vi "Calculation_Velocities_Statistics-3.vi"(8 "error IN":errorcluster, 9 "[IN] Velocities and Times":T3, 10 "[IN] Filtered Tracks":cluster{"Tracks":dbl[], "Start Pos":i32}[](array[cluster]), 11 "[IN] Movie Values":T2 {"Particle Fil Setups"."Type of particle filter"."Measurement Parameter" items=["Center of Mass X", "Center of Mass Y", "First Pixel X", "First Pixel Y", "Bounding Rect Left", "Bounding Rect Top", "Bounding Rect Right", "Bounding Rect Bottom", "Max Feret Diameter Start X", "Max Feret Diameter Start Y", "Max Feret Diameter End X", "Max Feret Diameter End Y", "Max Horiz. Segment Length Left", "Max Horiz. Segment Length Right", "Max Horiz. Segment Length Row", "-", "Bounding Rect Width", "Bounding Rect Height", "Bounding Rect Diagonal", "Perimeter", "Convex Hull Perimeter", "Holes' Perimeter", "Max Feret Diameter", "Equivalent Ellipse Major Axis", "Equivalent Ellipse Minor Axis", "Equivalent Ellipse Minor Axis (Feret)", "Equivalent Rect Long Side", "Equivalent Rect Short Side", "Equivalent Rect Diagonal", "Equivalent Rect Short Side (Feret)", "Average Horiz. Segment Length", "Average Vert. Segment Length", "Hydraulic Radius", "Waddel Disk Diameter", "-", "Area", "Holes' Area", "Particle & Holes' Area", "Convex Hull Area", "Image Area", "-", "Number of Holes", "Number of Horiz. Segments", "Number of Vert. Segments", "-", "Orientation", "Max Feret Diameter Orientation", "-", "% Area/Image Area", "% Area/(Particle & Holes' Area)", "Ratio of Equivalent Ellipse Axes", "Ratio of Equivalent Rect Sides", "-", "Elongation Factor", "Compactness Factor", "Heywood Circularity Factor", "Type Factor", "-", "Sum X", "Sum Y", "Sum XX", "Sum XY", "Sum YY", "Sum XXX", "Sum XXY", "Sum XYY", "Sum YYY", "-", "Moment of Inertia XX", "Moment of Inertia XY", "Moment of Inertia YY", "Moment of Inertia XXX", "Moment of Inertia XXY", "Moment of Inertia XYY", "Moment of Inertia YYY", "Norm. Moment of Inertia XX", "Norm. Moment of Inertia XY", "Norm. Moment of Inertia YY", "Norm. Moment of Inertia XXX", "Norm. Moment of Inertia XXY", "Norm. Moment of Inertia XYY", "Norm. Moment of Inertia YYY", "Hu Moment 1", "Hu Moment 2", "Hu Moment 3", "Hu Moment 4", "Hu Moment 5", "Hu Moment 6", "Hu Moment 7"]}) -> (0 "error OUT":errorcluster, 1 "[OUT] Velocities and Times":T3)   [LabVIEW 2013]
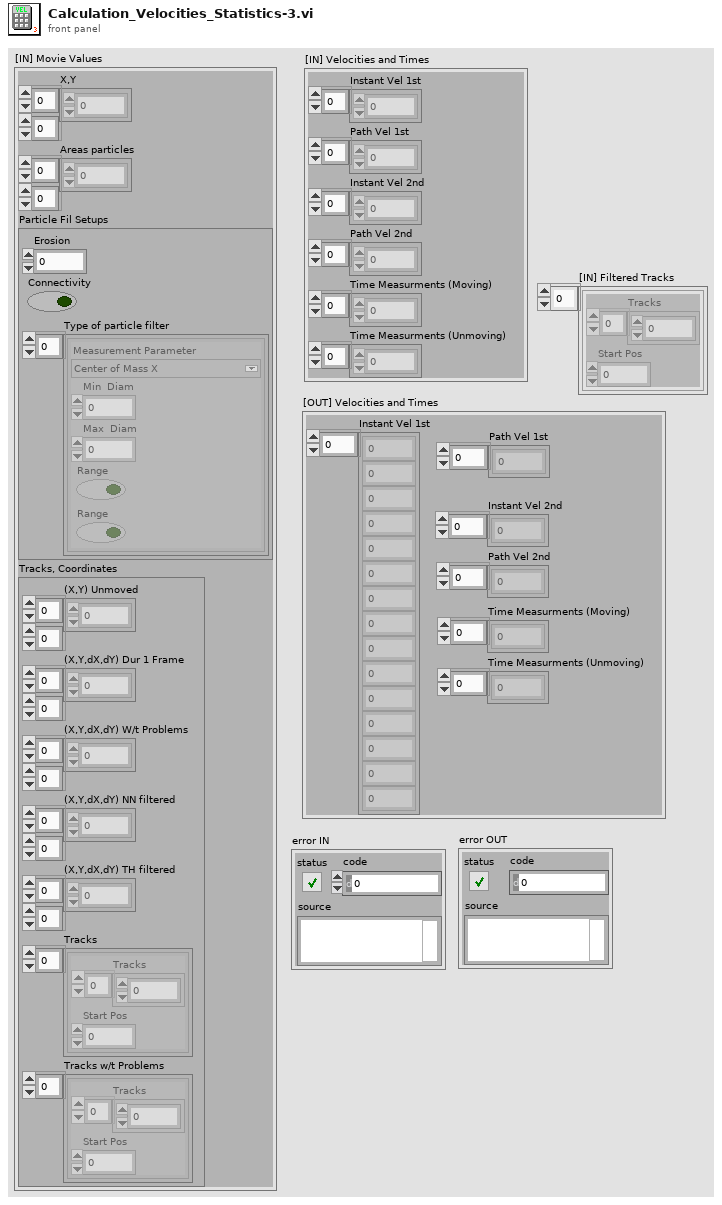
[diagram p1: front panel]
types:
  T1 = typedef "Particle Parameters" = i32
  T2 = cluster{"X,Y":dbl[][], "Areas particles":dbl[][], "Particle Fil Setups":cluster{"Erosion":i32, "Connectivity ":bool, "Type of particle filter":cluster{"Measurement Parameter":T1, "Min  Diam":dbl, "Max  Diam":dbl, "Range":bool, "Range":bool}[]}, "Tracks, Coordinates":cluster{"(X,Y) Unmoved":dbl[][], "(X,Y,dX,dY) Dur 1 Frame":dbl[][], "(X,Y,dX,dY) W/t Problems":dbl[][], "(X,Y,dX,dY) NN filtered":dbl[][], "(X,Y,dX,dY) TH filtered":dbl[][], "Tracks":cluster{"Tracks":dbl[], "Start Pos":i32}[], "Tracks w/t Problems":cluster{"Tracks":dbl[], "Start Pos":i32}[]}}
  T3 = cluster{"Instant Vel 1st":dbl[], "Path Vel 1st ":dbl[], "Instant Vel 2nd  ":dbl[], "Path Vel 2nd":dbl[], "Time Measurments (Moving)":i32[], "Time Measurments (Unmoving) ":i16[]}
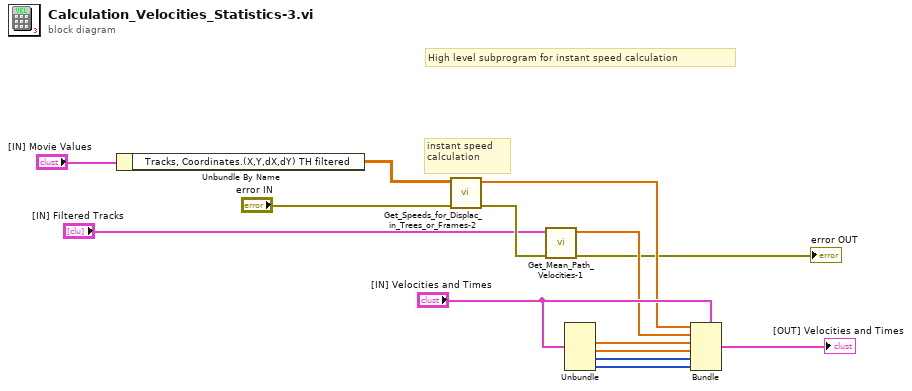
[diagram p0: block diagram]
diagram:
  # "High level subprogram for instant speed calculation"
  # "instant speed \ncalculation"
  n1 = Unbundle By Name("[IN] Movie Values") -> ("Tracks, Coordinates.(X,Y,dX,dY) TH filtered"=w2:dbl[][])
  n2 = call "Get_Speeds_for_Displac_in_Trees_or_Frames-2.vi"("error IN"="error IN", "[IN] Displacements in Frame-to-\nFrame Manner or in Tracks (Trees)"=w2) -> ("error OUT"=w6:errorcluster, "[OUT] Velocities\nin (pixel/frame)"=w8:dbl[])  [unwired: 4 in]
  n3 = call "Get_Mean_Path_Velocities-1.vi"("error IN"=w6, "[IN] Tracks + Starting Position"="[IN] Filtered Tracks") -> ("error OUT"=→"error OUT":errorcluster, "[OUT] Mean Path Velocities"=w5:dbl[])  [unwired: 4 in]
  n4 = Unbundle("[IN] Velocities and Times") -> ("Instant Vel 2nd"=w9:dbl[], "Path Vel 2nd"=w10:dbl[], "Time Measurments (Moving)"=w11:i32[], "Time Measurments (Unmoving)"=w12:i16[])  [unwired: 2 out]
  n5 = Bundle(cluster="[IN] Velocities and Times", "Instant Vel 1st"=w8, "Path Vel 1st"=w5, "Instant Vel 2nd"=w9, "Path Vel 2nd"=w10, "Time Measurments (Moving)"=w11, "Time Measurments (Unmoving)"=w12) -> (→"[OUT] Velocities and Times":T3)
